vi "FEED_Door_Status.vi"(11 "Array in":bool[](array[boolean])) -> (2 "Door Number":i32, 3 "Array out":bool[](array[boolean]))   [LabVIEW 2017]
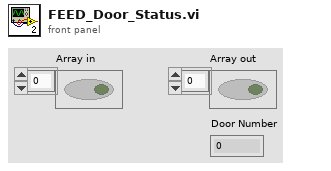
[diagram p1: front panel]
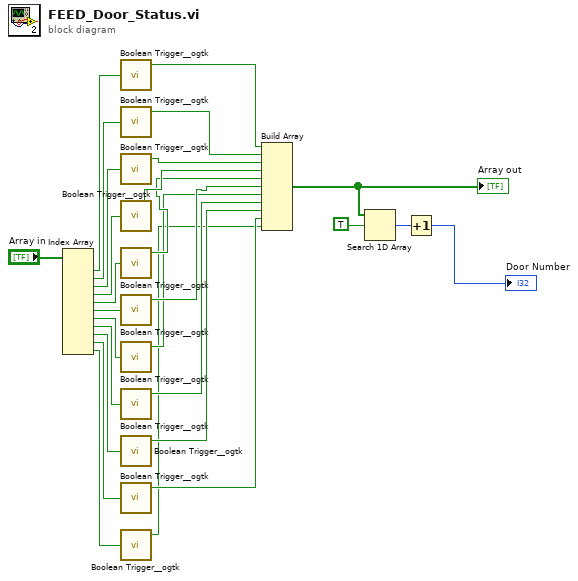
[diagram p0: block diagram]
diagram:
  n1 = Index Array(array="Array in") -> (element #1=w26:bool, element #2=w25:bool, element #3=w24:bool, element #4=w23:bool, element #5=w22:bool, element #6=w21:bool, element #7=w20:bool, element #8=w19:bool, element #9=w18:bool, element #10=w17:bool, element #11=w16:bool)  [unwired: 11 in]
  n2 = call <userlib>:"Boolean Trigger__ogtk.vi"("Boolean Input"=w26) -> ("Rising Edge"=w15:bool)  [unwired: 1 in, 1 out]
  n3 = call <userlib>:"Boolean Trigger__ogtk.vi"("Boolean Input"=w25) -> ("Rising Edge"=w14:bool)  [unwired: 1 in, 1 out]
  n4 = call <userlib>:"Boolean Trigger__ogtk.vi"("Boolean Input"=w24) -> ("Rising Edge"=w13:bool)  [unwired: 1 in, 1 out]
  n5 = call <userlib>:"Boolean Trigger__ogtk.vi"("Boolean Input"=w23) -> ("Rising Edge"=w12:bool)  [unwired: 1 in, 1 out]
  n6 = call <userlib>:"Boolean Trigger__ogtk.vi"("Boolean Input"=w22) -> ("Rising Edge"=w11:bool)  [unwired: 1 in, 1 out]
  n7 = call <userlib>:"Boolean Trigger__ogtk.vi"("Boolean Input"=w21) -> ("Rising Edge"=w10:bool)  [unwired: 1 in, 1 out]
  n8 = call <userlib>:"Boolean Trigger__ogtk.vi"("Boolean Input"=w20) -> ("Rising Edge"=w9:bool)  [unwired: 1 in, 1 out]
  n9 = call <userlib>:"Boolean Trigger__ogtk.vi"("Boolean Input"=w19) -> ("Rising Edge"=w8:bool)  [unwired: 1 in, 1 out]
  n10 = call <userlib>:"Boolean Trigger__ogtk.vi"("Boolean Input"=w18) -> ("Rising Edge"=w7:bool)  [unwired: 1 in, 1 out]
  n11 = call <userlib>:"Boolean Trigger__ogtk.vi"("Boolean Input"=w17) -> ("Rising Edge"=w6:bool)  [unwired: 1 in, 1 out]
  n12 = call <userlib>:"Boolean Trigger__ogtk.vi"("Boolean Input"=w16) -> ("Rising Edge"=w5:bool)  [unwired: 1 in, 1 out]
  n13 = Build Array(w15, w14, w13, w12, w11, w10, w9, w8, w7, w6, w5) -> (w4:bool[])
  "Array out" <- w4
  n14 = Search 1D Array(1D array=w4, element=TRUE) -> (index of element=w2:i32)  [unwired: 1 in]
  n15 = Increment(x=w2) -> (x+1=→"Door Number":i32)
